vi "Configure Sweep.vi"   [LabVIEW 2012, in "Agilent PSG MXG Series.lvlib"]
doc: "Configures list, step and ramp sweep."
uses:
  <instrlib>/Agilent PSG MXG Series/Agilent PSG MXG Series.lvlib
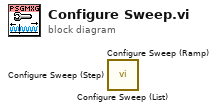
[diagram p0: block diagram]
diagram:
  n1 = call <instrlib>:"Configure Sweep (List).vi"() -> ()  [unwired: 14 in, 2 out]
  n2 = call <instrlib>:"Configure Sweep (Ramp).vi"() -> ()  [unwired: 14 in, 2 out]
  n3 = call <instrlib>:"Configure Sweep (Step).vi"() -> ()  [unwired: 14 in, 2 out]
